vi "Emergency_stop_and_Reset.vi"() -> ()   [LabVIEW 2017]
panel:
  out "E-Stop status":picture
  out "Response time":u32
  out "Test Result status":picture
  out "XY Graph":cluster{dbl, u32}[](graph)
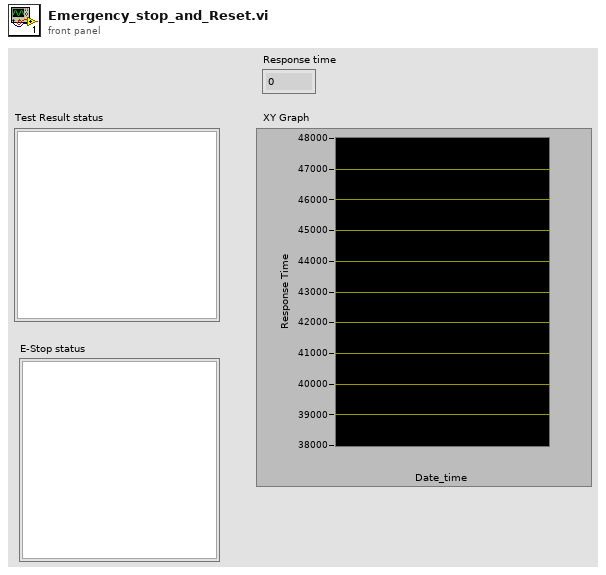
[diagram p1: front panel]
types:
  T1 = enum16{"open", "replace", "create", "open or create", "replace or create", "replace or create with confirmation"}
  T2 = cluster{"[0]":string, "[1]":string, "[2]":string, "[3]":string, "[4]":string, "[5]":string, "[6]":string, "[7]":string, "[8]":string}
  T3 = cluster{"Iterations":u32, "DelayBetweenIterations":u32, "Timeout":u32, "USB6008Port":string, "ActiveLow":i32, "DelayToResetEstop":i32, "ActiveHigh":i32, "Trigger_source":string, "SamplesRate":i32, "Timestamp":string, "TestSuite":string, "ReportPath":path, "FWVersionPath":path}
  T4 = cluster{"Socket_IP_Address":string, "Socket_Port_Number":u16, "Global_ReportPath":path}
  T5 = typedef "imagedata.ctl" = cluster{"image type":i32, "image depth":i32, "image":u8[], "mask":u8[], "colors":u32[], "Rectangle":cluster{"left":i16, "top":i16, "right":i16, "bottom":i16}}
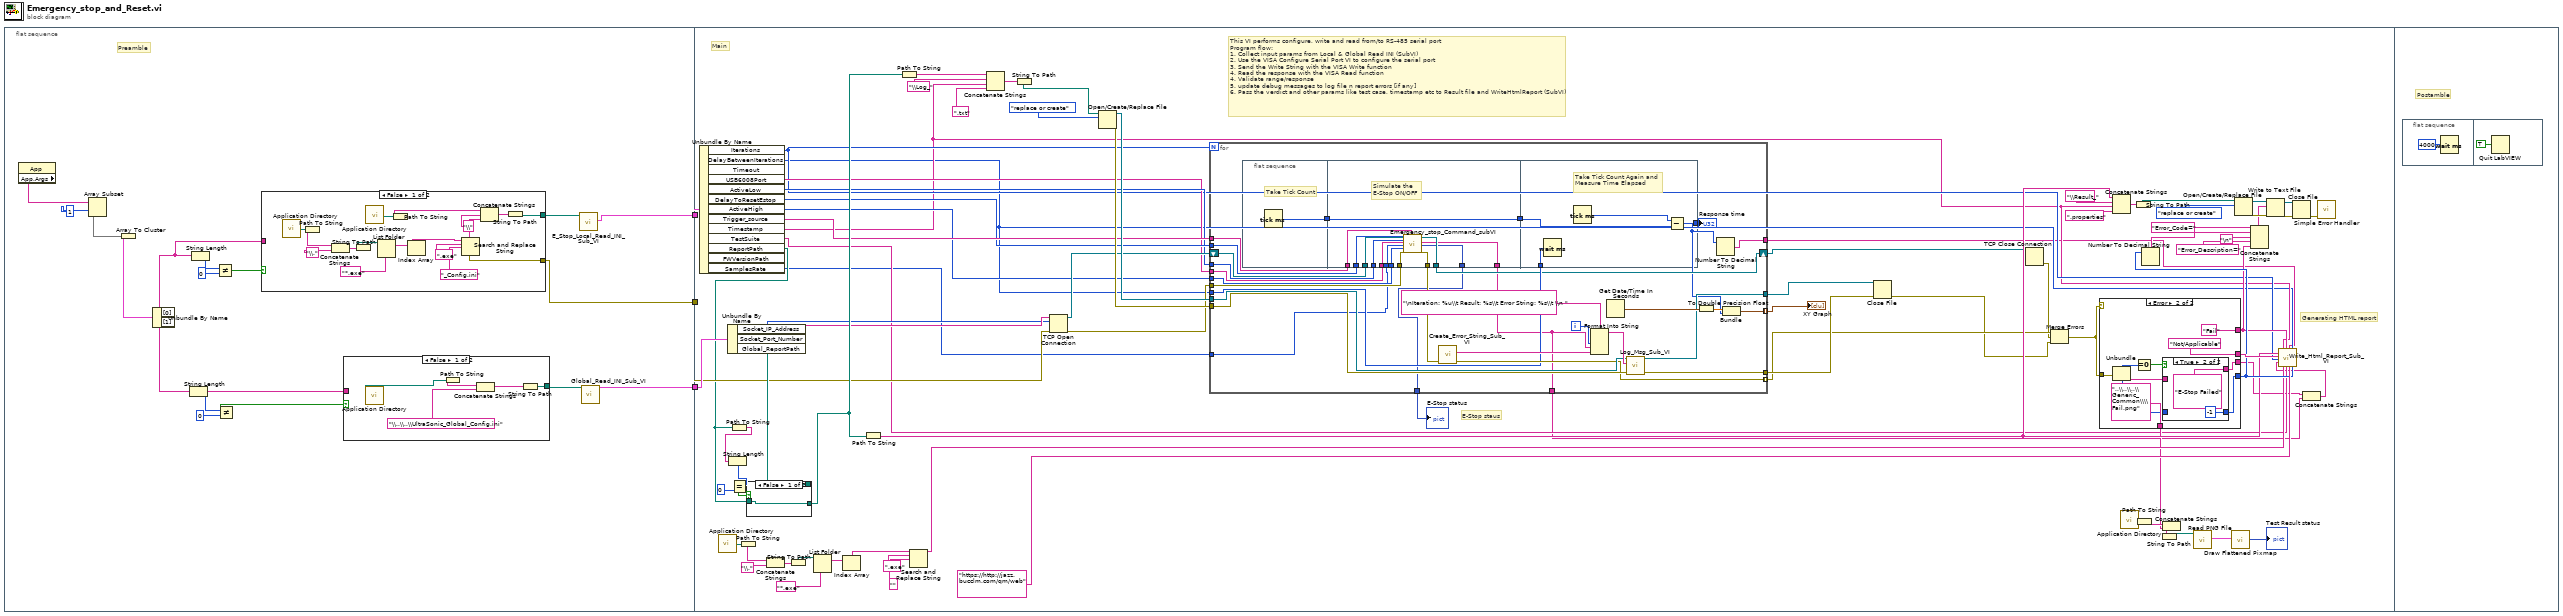
[diagram p0: block diagram]
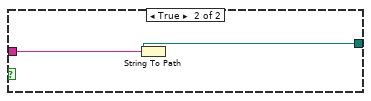
[diagram p2: hidden frame]
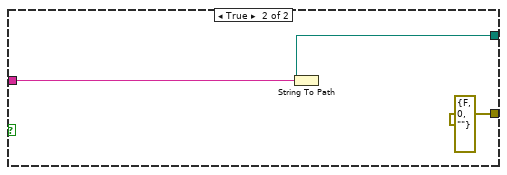
[diagram p3: hidden frame]
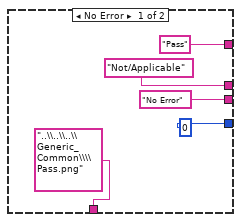
[diagram p5: hidden frame]
diagram:
  n1 = flat-sequence {
    tunnel: [w6] -> w3
    tunnel: [w5] -> w2
    tunnel: [w4] -> w1
    tunnel: w3 -> [w70]
    tunnel: w2 -> [w75]
    tunnel: w1 -> [w65]
    frame #0 {
      # "Preamble"
      n2 = property class="App"() -> ("App.Args"=w8:string[])  [unwired: 2 in, 2 out]
      n3 = Array Subset "Array Subset"(array=w8, index=1) -> (w9:string[])  [unwired: 1 in]
      n4 = Array To Cluster(array=w9) -> (cluster=w10:T2)
      n5 = Unbundle By Name "Unbundle By Name"(w10) -> ("[0]"=w14:string, "[1]"=w17:string)
      n6 = String Length(string=w17) -> (length=w18:i32)
      n7 = String Length(string=w14) -> (length=w11:i32)
      n8 = Not Equal?(x=w11, y=0) -> (x != y?=w13:bool)
      n9 = Not Equal?(x=w18, y=0) -> (x != y?=w16:bool)
      n10 = case shown="False" w13 {
        tunnel: w14 -> [_ w47]
        tunnel: [w29 w46] -> w19
        tunnel: [w28 errorcluster {"status"=FALSE, "code"=0, "source"=""} ("error out")] -> w6
        frame False {
          n11 = call <vilib>:"Application Directory.vi"() -> ("Application Directory"=w35:path)
          n12 = Path To String(path=w35) -> (string=w34:string)
          n13 = Concatenate Strings(w34, "\\." ("string")) -> (w32:string)
          n14 = String To Path(string=w32) -> (path=w37:path)
          n15 = call <vilib>:"Application Directory.vi"() -> ("Application Directory"=w44:path)
          n16 = List Folder(path=w37, pattern="*.exe") -> (filenames=w31:string[])  [unwired: 2 in, 3 out]
          n17 = Path To String(path=w44) -> (string=w39:string)
          n18 = Index Array(array=w31) -> (element=w30:string)  [unwired: 1 in]
          n19 = Search and Replace String(input string=w30, search string=".exe", replace string="_Config.ini" ("replace string (\"\")")) -> (result string=w41:string, error out=w28:errorcluster)  [unwired: 5 in, 2 out]
          n20 = Concatenate Strings(w39, "\\" ("string"), w41) -> (w38:string)
          n21 = String To Path(string=w38) -> (path=w29:path)
        }
        frame True {
          n22 = String To Path(string=w47) -> (path=w46:path)
        }
      }
      n23 = case shown="False" w16 {
        tunnel: [w22 w27] -> w20
        tunnel: w17 -> [_ w26]
        frame False {
          n24 = call <vilib>:"Application Directory.vi"() -> ("Application Directory"=w21:path)
          n25 = Path To String(path=w21) -> (string=w25:string)
          n26 = Concatenate Strings(w25, "\\..\\..\\UltraSonic_Global_Config.ini" ("string")) -> (w23:string)
          n27 = String To Path(string=w23) -> (path=w22:path)
        }
        frame True {
          n28 = String To Path(string=w26) -> (path=w27:path)
        }
      }
      n29 = call "E_Stop_Local_Read_INI_Sub_VI.vi"("Config File Path"=w19) -> ("E-stop Parameters"=w4:T3)  [unwired: 10 in]
      n30 = call "Global_Read_INI_Sub_VI.vi"("Config File Path"=w20) -> ("output cluster"=w5:T4)  [unwired: 14 in]
    }
    frame #1 {
      # "Generating HTML report"
      # "E-Stop staus"
      # "This VI performs configure, write and read from/to RS-485 serial port\nProgram flow:\n1. Collect input params from Local & Global Read INI (SubVI)\n2. Use the VISA Configure Serial Port VI to configure the serial port\n3. Send the Write String with the VISA Write function\n4. Read the response with the VISA Read function\n4. Validate range/response\n5. update debug messages to log file n report errors [if any]\n6. Pass the verdict and other params like test case, timestamp etc to Result file and WriteHtmlReport (SubVI)"
      # "Main"
      n31 = Unbundle By Name(w65) -> ("Iterations"=w51:u32, "DelayBetweenIterations"=w49:u32, "USB6008Port"=w61:string, "ActiveLow"=w62:i32, "DelayToResetEstop"=w63:i32, "ActiveHigh"=w60:i32, "Trigger_source"=w64:string, "Timestamp"=w50:string, "TestSuite"=w58:string, "ReportPath"=w59:path, "SamplesRate"=w57:i32)  [unwired: 2 out]
      n32 = call <vilib>:"Application Directory.vi"() -> ("Application Directory"=w91:path)
      n33 = Unbundle By Name(w75) -> ("Socket_IP_Address"=w72:string, "Socket_Port_Number"=w71:u16, "Global_ReportPath"=w74:path)
      n34 = Path To String(path=w59) -> (string=w122:string)
      n35 = String Length(string=w122) -> (length=w121:i32)
      n36 = Equal?(x=w121, y=0) -> (x = y?=w119:bool)
      n37 = Path To String(path=w91) -> (string=w90:string)
      n38 = case shown="False" w119 {
        tunnel: w74 -> [_ w132]
        tunnel: [w131 w132] -> w118
        tunnel: w59 -> [w131 _]
        frame False {
        }
        frame True {
        }
      }
      n39 = Concatenate Strings(w90, "\\." ("string")) -> (w88:string)
      n40 = String To Path(string=w88) -> (path=w93:path)
      n41 = List Folder(path=w93, pattern="*.exe") -> (filenames=w87:string[])  [unwired: 2 in, 3 out]
      n42 = Index Array(array=w87) -> (element=w83:string)  [unwired: 1 in]
      n43 = Path To String(path=w118) -> (string=w95:string)
      n44 = Path To String(path=w118) -> (string=w124:string)
      n45 = Search and Replace String(input string=w83, search string=".exe", replace string="" ("replace string (\"\")")) -> (result string=w86:string)  [unwired: 5 in, 3 out]
      n46 = Concatenate Strings(w124, "\\Log_" ("string"), w50, ".txt" ("string")) -> (w127:string)
      n47 = String To Path(string=w127) -> (path=w126:path)
      n48 = TCP Open Connection(address=w72, remote port or service name=w71, error in (no error)=w70) -> (connection ID=w66:refnum<k5>, error out=w69:errorcluster)  [unwired: 2 in]
      n49 = Open/Create/Replace File(file path (use dialog)=w126, operation (0:open)=T1."replace or create") -> (refnum out=w96:refnum<file>, error out=w99:errorcluster)  [unwired: 1 in, 4 out]
      n50 = for {
        N: w51 -> [_]
        tunnel: w96 -> [w156]
        tunnel: [w155] -> w98
        tunnel: [w153] -> w97
        tunnel: [w158] -> w128 mode=indexing
        tunnel: w99 -> [w154]
        tunnel: [w151] -> w94 mode=indexing
        tunnel: w69 -> [w140]
        shift-right: [w138] -> w67
        shift-left: w66 -> [w146]
        tunnel: w49 -> [w149]
        tunnel: w64 -> [w145]
        tunnel: w63 -> [w144]
        tunnel: w62 -> [w143]
        tunnel: w61 -> [w142]
        tunnel: w60 -> [w141]
        tunnel: w57 -> [w137]
        tunnel: [w136] -> w55
        tunnel: [w135] -> w53
        tunnel: [w133] -> w48
        i -> [w152]
        n51 = flat-sequence {
          tunnel: [w162] -> w148
          tunnel: w148 -> [w175]
          tunnel: [w175] -> w147
          tunnel: w146 -> [w174]
          tunnel: w145 -> [w173]
          tunnel: w144 -> [w172]
          tunnel: w143 -> [w171]
          tunnel: w142 -> [w170]
          tunnel: w141 -> [w169]
          tunnel: w140 -> [w168]
          tunnel: [w167] -> w139
          tunnel: [w166] -> w138
          tunnel: [w165] -> w135
          tunnel: w137 -> [w164]
          tunnel: [w163] -> w136
          tunnel: w147 -> [w179]
          tunnel: [w177] -> w134
          tunnel: w149 -> [w176]
          frame #0 {
            # "Take Tick Count"
            n52 = Tick Count (ms)() -> (millisecond timer value=w162:u32)
          }
          frame #1 {
            # "Simulate the \nE-Stop ON/OFF"
            n53 = call "Emergency_stop_Command_subVI.vi"("TCP connection ID IN"=w174, "Active Low"=w171, "Port"=w170, "Rate"=w164, "dioHigh"=w169, "ERROR IN"=w168, "Delay to reset e-stop"=w172, "Trigger Source"=w173) -> ("TCP Connection \nID out"=w166:refnum<k5>, "E-Stop output"=w165:string, "Estop Test Result"=w163:picture, "ERROR OUT"=w167:errorcluster)  [unwired: 8 in]
          }
          frame #2 {
            # "Take Tick Count Again and Measure Time Elapsed"
            n54 = Wait (ms)(milliseconds to wait=w176) -> ()  [unwired: 1 out]
            n55 = Tick Count (ms)() -> (millisecond timer value=w178:u32)
            n56 = Subtract(x=w178, y=w179) -> (x-y=w177:u32)
          }
        }
        n57 = call "Create_Error_String_Sub_VI.vi"("error in"=w139) -> ("error out"=w151:errorcluster, "Error String"=w150:string)  [unwired: 9 in]
        n58 = Format Into String(format string="\nIteration: %u\\t Result: %s\\t Error String: %s\\t \\n ", w152, w135, w150) -> (resulting string=w157:string)  [unwired: 2 in, 1 out]
        n59 = Get Date/Time In Seconds() -> (seconds since 1Jan1904=w159:timestamp)
        n60 = call "Log_Msg_Sub_VI.vi"("error in (no error)"=w154, "String"=w157, "Byte Stream File in"=w156) -> ("error out"=w153:errorcluster, "Byte Stream File out"=w155:refnum<file>)  [unwired: 7 in]
        n61 = To Double Precision Float(number=w159) -> (double precision float=w160:dbl)
        n62 = Number To Decimal String(number=w134) -> (decimal integer string=w133:string)  [unwired: 1 in]
        n63 = Bundle "Bundle"(w160, w134) -> (w158:cluster{dbl, u32})  [unwired: 1 in]
        "Response time" <- w134
      }
      "XY Graph" <- w128
      "E-Stop status" <- w55
      n64 = Close File(refnum=w98, error in=w97) -> (error out=w56:errorcluster)  [unwired: 1 out]
      n65 = TCP Close Connection(connection ID=w67) -> (error out=w68:errorcluster)  [unwired: 2 in, 1 out]
      n66 = Merge Errors "Merge Errors"(w94, w68, w56) -> (w73:errorcluster)
      n67 = case shown="Error" w73 {
        tunnel: ["Pass" "Fail"] -> w100
        tunnel: w73 -> [_ w191]
        tunnel: [0 ("code") w187] -> w104
        tunnel: ["No Error" ("source") w188] -> w54
        tunnel: ["Not/Applicable" "Not/Applicable"] -> w130
        tunnel: ["..\\..\\..\\Generic_Common\\\\Pass.png" ("string") "..\\..\\..\\Generic_Common\\\\Fail.png" ("string")] -> w76
        frame No Error {
        }
        frame Error {
          n68 = Unbundle(w191) -> ("code"=w189:i32, "source"=w185:string)  [unwired: 1 out]
          n69 = Equal To 0?(x=w189) -> (x = 0?=w186:bool)
          n70 = case shown="True" w186 {
            tunnel: [w195 -1 ("code")] -> w187
            tunnel: [w194 "E-Stop Failed" ("source")] -> w188
            tunnel: w189 -> [w195 _]
            tunnel: w185 -> [w194 _]
            frame False {
            }
            frame True {
            }
          }
        }
      }
      n71 = Concatenate Strings(w95, "\\Result_" ("string"), w50, ".properties" ("string")) -> (w116:string)
      n72 = call <vilib>:"Application Directory.vi"() -> ("Application Directory"=w77:path)
      n73 = String To Path(string=w116) -> (path=w108:path)
      n74 = Path To String(path=w77) -> (string=w78:string)
      n75 = Number To Decimal String(number=w104) -> (decimal integer string=w103:string)  [unwired: 1 in]
      n76 = Concatenate Strings(w78, w76) -> (w79:string)
      n77 = String To Path(string=w79) -> (path=w82:path)
      n78 = call <vilib>:"Read PNG File.vi"("path to PNG file"=w82) -> ("image data"=w80:T5)  [unwired: 8 in, 2 out]
      n79 = call <vilib>:"Draw Flattened Pixmap.vi"("image data"=w80) -> ("new picture"=→"Test Result status":picture)  [unwired: 8 in]
      n80 = Open/Create/Replace File(file path (use dialog)=w108, operation (0:open)=T1."replace or create") -> (refnum out=w107:refnum<file>, error out=w112:errorcluster)  [unwired: 4 in, 1 out]
      n81 = Concatenate Strings("Error_Code=" ("string"), w103, "\n", "Error_Description=" ("string"), w100) -> (w106:string)
      n82 = Write to Text File(file (use dialog)=w107, text=w106, error in=w112) -> (refnum out=w111:refnum<file>, error out=w110:errorcluster)  [unwired: 1 in, 1 out]
      n83 = Close File(refnum=w111, error in=w110) -> (error out=w109:errorcluster)  [unwired: 1 out]
      n84 = Concatenate Strings(w54, w53) -> (w52:string)
      n85 = call "Write_Html_Report_Sub_VI.vi"("ReprtPath"=w95, "Remarks"=w130, "Iterations"=w51, "Error Description"=w52, "Timestamp"=w50, "TestCase"=w86, "Verdict"=w100, "TestSuite"=w58, "Time taken to execute  test in msec"=w48, "JazzDashboardLink"="https://http://jazz.bucclm.com/qm/web" ("TestSuite"), "Delay Between Iterations"=w49, "Error Code"=w104) -> ()  [unwired: 8 in]
      n86 = call <vilib>:"Simple Error Handler.vi"("error in (no error)"=w109) -> ()  [unwired: 4 in, 5 out]
    }
    frame #2 {
      # "Postamble"
      n87 = flat-sequence {
        frame #0 {
          n88 = Wait (ms)(milliseconds to wait=u32 4000) -> ()  [unwired: 1 out]
        }
        frame #1 {
          n89 = Quit LabVIEW(quit? (T)=TRUE) -> ()
        }
      }
    }
  }
